vi "ma_Locate three fingers of single tone (FFT input, CDB).vi"(8 "advanced search":T2={"approx freq. (optional)"=nan, "search (+/- % of Fsampl.)"=5.0} {"search (+/- % of Fsampl.)" format="%0.2p"; "approx freq. (optional)" format="%0.2p"}, 9 "fs":dbl, 10 "FFT size":i32, 11 "Complex  Hann spectrum":cdb[](array[numeric])) -> (3 "three fingers":T1={"f0"=0.0, "df"=1.0, "spectrum"=[]} {"spectrum" format="%.2f"; "df" format="%.2f"; "f0" format="%.2f"})   [LabVIEW 2020, in "NI_MAPro.lvlib"]
uses:
  NI_MAPro.lvlib
  ma_sml_Spectrum Cluster (complex).ctl
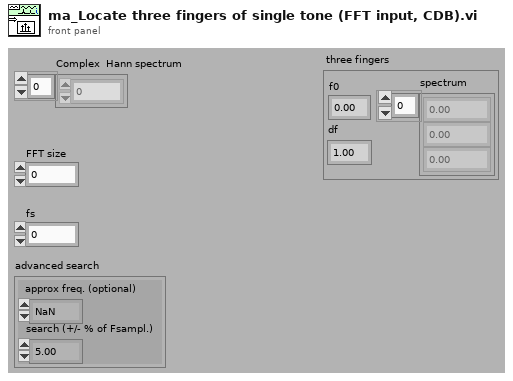
[diagram p1: front panel]
types:
  T1 = typedef "NI_MAPro.lvlib/ma_sml_Spectrum Cluster (complex).ctl" = cluster{"f0":dbl, "df":dbl, "spectrum":cdb[]}
  T2 = cluster{"approx freq. (optional)":dbl, "search (+/- % of Fsampl.)":dbl}
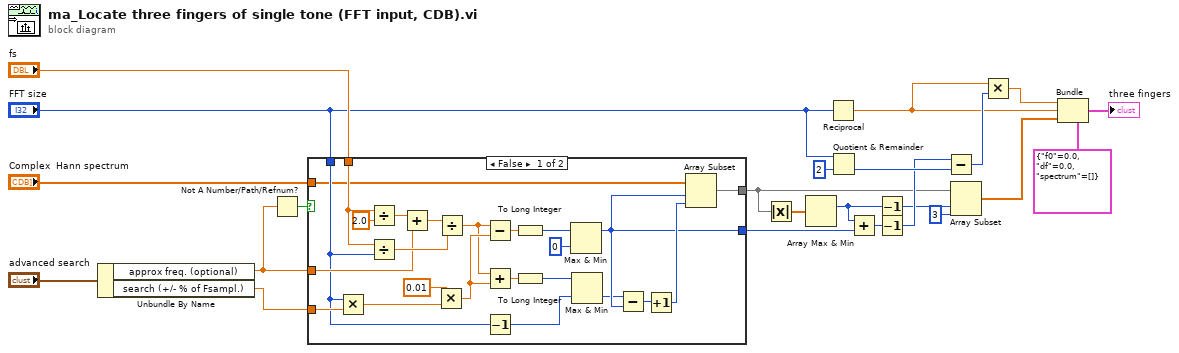
[diagram p0: block diagram]
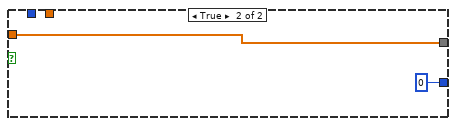
[diagram p2: hidden frame]
diagram:
  n1 = Unbundle By Name("advanced search") -> ("approx freq. (optional)"=w12:dbl, "search (+/- % of Fsampl.)"=w9:dbl)
  n2 = Not A Number/Path/Refnum?(number/path/refnum=w12) -> (NaN/Path/Refnum?=w14:bool)
  n3 = case shown="False" w14 {
    tunnel: "Complex  Hann spectrum" -> [w29 w49]
    tunnel: [w26 w49] -> w1
    tunnel: w12 -> [w42 _]
    tunnel: "fs" -> [w43 _]
    tunnel: "FFT size" -> [w31 _]
    tunnel: w9 -> [w41 _]
    tunnel: [w25 0] -> w8
    frame False {
      n4 = Multiply(x=w31, y=w41) -> (x*y=w40:dbl)
      n5 = Divide(x=w43, y=2.0) -> (x/y=w45:dbl)
      n6 = Divide(x=w43, y=w31) -> (x/y=w47:dbl)
      n7 = Add(x=w45, y=w42) -> (x+y=w46:dbl)
      n8 = Multiply(x=0.01, y=w40) -> (x*y=w38:dbl)
      n9 = Divide(x=w46, y=w47) -> (x/y=w37:dbl)
      n10 = Subtract(x=w37, y=w38) -> (x-y=w36:dbl)
      n11 = Add(x=w37, y=w38) -> (x+y=w35:dbl)
      n12 = Decrement(x=w31) -> (x-1=w30:i32)
      n13 = To Long Integer(number=w36) -> (32bit integer=w34:i32)
      n14 = To Long Integer(number=w35) -> (32bit integer=w32:i32)
      n15 = Max & Min(x=w34, y=0) -> (max(x,y)=w25:i32)  [unwired: 1 out]
      n16 = Max & Min(x=w32, y=w30) -> (min(x,y)=w24:i32)  [unwired: 1 out]
      n17 = Subtract(x=w24, y=w25) -> (x-y=w28:i32)
      n18 = Increment(x=w28) -> (x+1=w27:i32)
      n19 = Array Subset(array=w29, index=w25, length=w27) -> (w26:cdb[])
    }
    frame True {
    }
  }
  n20 = Absolute Value(x=w1) -> (abs(x)=w2:dbl[])
  n21 = Array Max & Min(array=w2) -> (max index (indices)=w4:i32)  [unwired: 3 out]
  n22 = Reciprocal(x="FFT size") -> (1/x=w18:dbl)
  n23 = Quotient & Remainder(x="FFT size", y=2) -> (floor(x/y)=w21:i32)  [unwired: 1 out]
  n24 = Add(x=w4, y=w8) -> (x+y=w5:i32)
  n25 = Decrement(x=w4) -> (x-1=w3:i32)
  n26 = Decrement(x=w5) -> (x-1=w7:i32)
  n27 = Subtract(x=w7, y=w21) -> (x-y=w23:i32)
  n28 = Array Subset(array=w1, index=w3, length=3) -> (w16:cdb[])
  n29 = Multiply(x=w18, y=w23) -> (x*y=w17:dbl)
  n30 = Bundle(cluster=T1 {"f0"=0.0, "df"=0.0, "spectrum"=[]} ("FFT spectrum 2"), "f0"=w17, "df"=w18, "spectrum"=w16) -> (→"three fingers":T1)
